vi "DefineColorPalette.vi"(10 "Files in":T2[](array[typedef]), 11 "FileList":refnum<vi>) -> (2 "Files out":T2[](array[typedef]))   [LabVIEW 2022 SP3]
uses:
  Curtin1_Label.ctl
panel:
  in  "new name":T1
  in  "Delete":bool
  in  "Clear":bool
  in  "Save":bool
  in  "Save as":bool
  in  "Apply":bool
  in  "Your Color Palettes":u16(ring) items=["Last Saved", "24 Colors", "fred", "rear"]
  in  "Colors":u32[](array[colorbox])
  # "Enter Color Name"
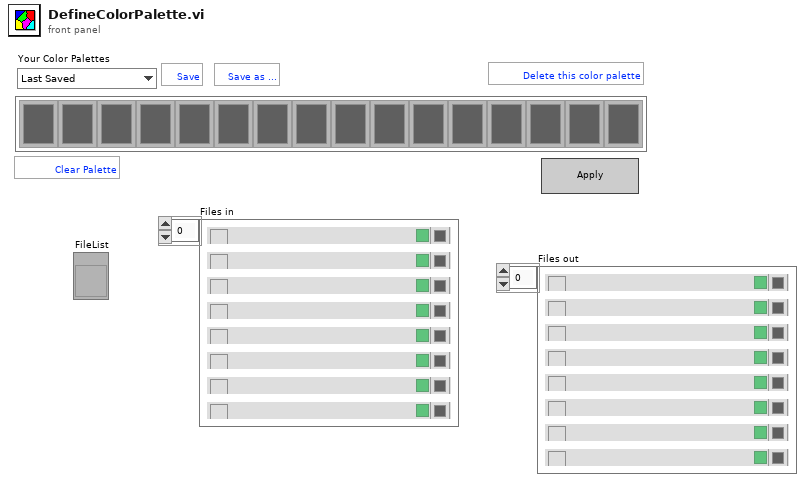
[diagram p1: front panel]
types:
  T1 = cluster{"Color Name":string, "OK Button":bool, "Cancel Button":bool}
  T2 = typedef "Curtin1_Label.ctl" = cluster{"Show?":bool, "Name":string, "Color":u32, "Path":path, "Show Notes":bool, "correlate":bool}
  T3 = enum16{"big-endian, network order", "native, host order", "little-endian"}
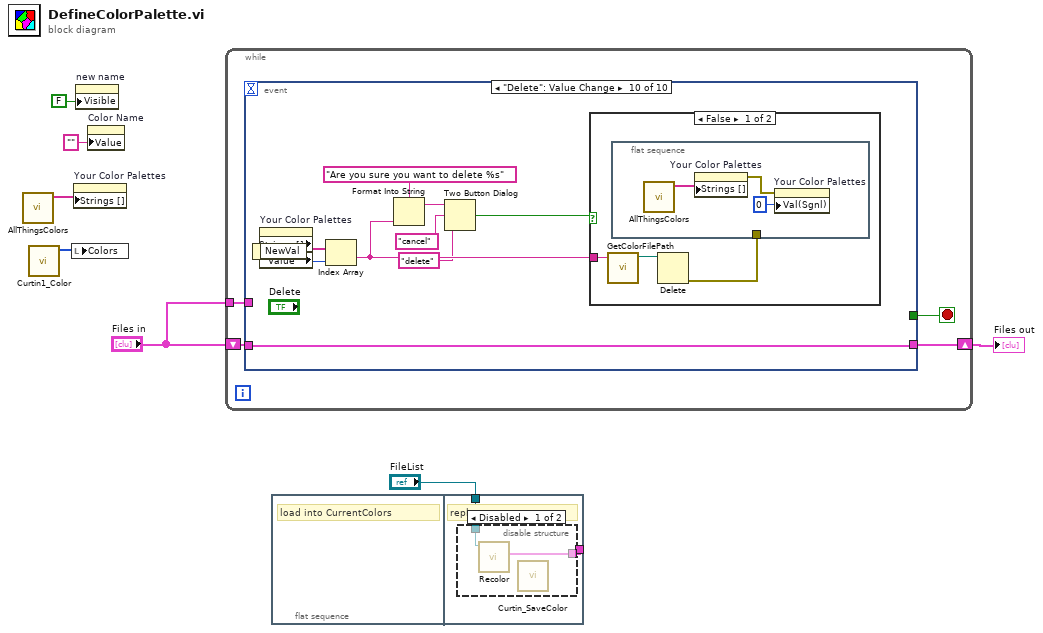
[diagram p0: block diagram]
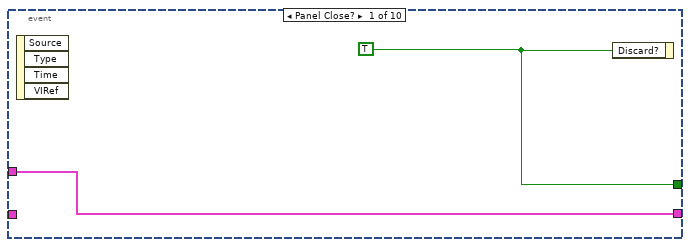
[diagram p3: hidden frame]
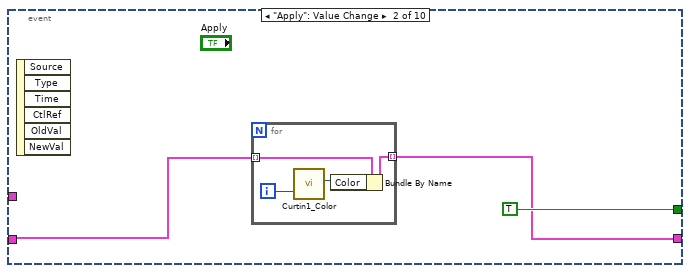
[diagram p4: hidden frame]
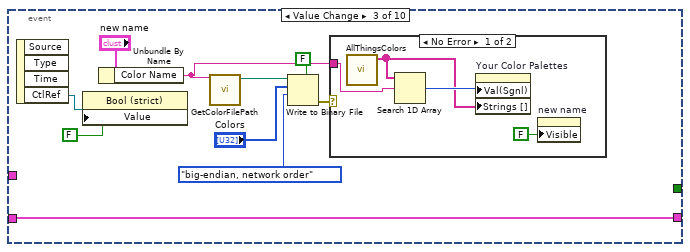
[diagram p5: hidden frame]
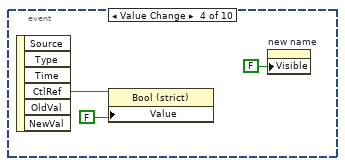
[diagram p7: hidden frame]
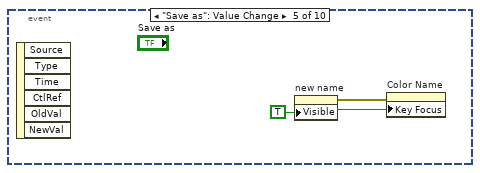
[diagram p8: hidden frame]
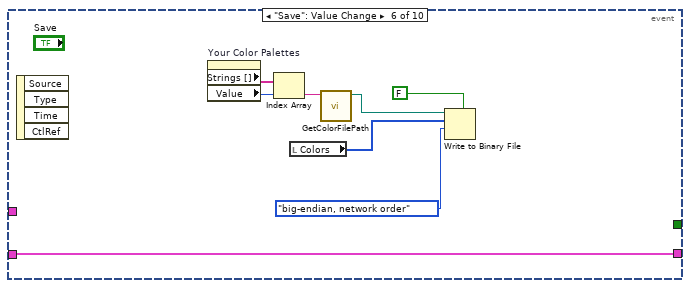
[diagram p9: hidden frame]
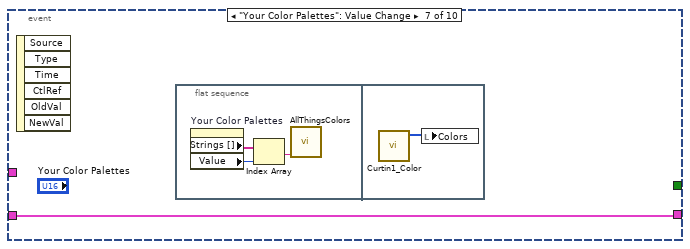
[diagram p10: hidden frame]
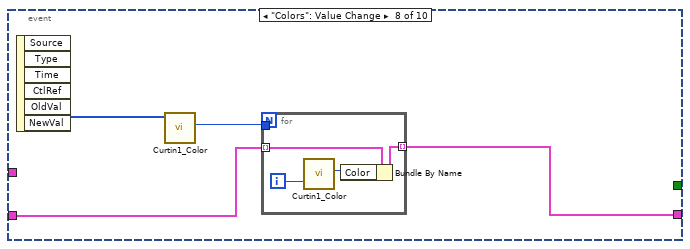
[diagram p11: hidden frame]
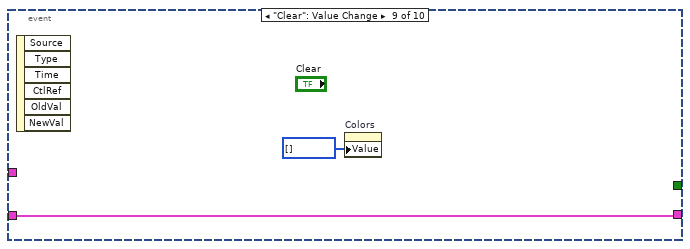
[diagram p12: hidden frame]
diagram:
  n1 = call "AllThingsColors.vi"() -> ("Possible Colors"=w7:string[])  [unwired: 11 in]
  n2 = call "Curtin1_Color.vi"() -> ("Color palette"=w3:u32[])  [unwired: 10 in, 1 out]
  n3 = local write "Colors"(w3) -> ()
  n4 = property on="Your Color Palettes" class="Ring (strict)"("Strings []"=w7) -> ()  [unwired: 2 in, 2 out]
  n5 = property on="new name" class="Clust (strict)"("Visible"=FALSE) -> ()  [unwired: 2 in, 2 out]
  n6 = property on="Color Name" class="Str"("Value"="") -> ()  [unwired: 2 in, 2 out]
  n7 = while {
    shift-right: [w10] -> w6
    shift-left: "Files in" -> [w9]
    tunnel: "Files in" -> [w8]
    stop <- w11 stop-if-true
    n8 = event shown="[9] \"Delete\": Value Change" {
      selector: _ -> [_ _ _ _ _ _ _ _ _ _]
      dyn-events: _ -> [_ _ _ _ _ _ _ _ _ _]
      timeout: _ -> [_ _ _ _ _ _ _ _ _ _]
      tunnel: [w13 TRUE ("Discard?") _ _ _ _ _ _ _ _] -> w11
      tunnel: [w12 w15 w30 _ _ w47 w48 w54 w62 w71] -> w10
      tunnel: w9 -> [_ w14 w30 _ _ w47 w48 w55 w62 w71]
      tunnel: w8 -> [w12 _ _ _ _ _ _ _ _ _]
      event Panel Close? {
        w13 = TRUE ("Discard?")
        n9 = event-data() -> ()  [unwired: 1 in, 4 out]
        n10 = event-data("Discard?"=w13) -> ()  [unwired: 1 in, 1 out]
      }
      event "Apply": Value Change {
        n11 = event-data() -> ()  [unwired: 1 in, 6 out]
        n12 = for {
          tunnel: w14 -> [w20] mode=indexing
          tunnel: [w19] -> w15 mode=indexing
          i -> [w18]
          n13 = call "Curtin1_Color.vi"("Offset"=w18) -> ("New color"=w17:u32)  [unwired: 9 in, 1 out]
          n14 = Bundle By Name(cluster=w20, "Color"=w17) -> (w19:T2)
        }
      }
      event "new name.OK Button": Value Change {
        n15 = event-data() -> ("CtlRef"=w21:refnum<vi>)  [unwired: 1 in, 3 out]
        n16 = property class="Bool (strict)"(reference=w21, "Value"=FALSE ("Visible")) -> ()  [unwired: 1 in, 2 out]
        n17 = Unbundle By Name("new name") -> ("Color Name"=w23:string)
        n18 = call "GetColorFilePath.vi"("String"=w23) -> ("path"=w25:path)  [unwired: 9 in, 1 out]
        n19 = Write to Binary File(file (use dialog)=w25, data="Colors", 5:FALSE ("prepend array or string size? (T)"), 9:T3."big-endian, network order" ("byte order (0:big-endian, network order)")) -> (error out=w26:errorcluster)  [unwired: 2 in, 2 out]
        n20 = case shown="No Error" w26 {
          tunnel: w23 -> [w34 _]
          frame No Error {
            n21 = call "AllThingsColors.vi"() -> ("Possible Colors"=w32:string[])  [unwired: 11 in]
            n22 = Search 1D Array(1D array=w32, element=w34) -> (index of element=w33:i32)  [unwired: 1 in]
            n23 = property on="Your Color Palettes" class="Ring (strict)"("Val(Sgnl)"=w33, "Strings []"=w32) -> ()  [unwired: 2 in, 2 out]
            n24 = property on="new name" class="Clust (strict)"("Visible"=FALSE) -> ()  [unwired: 2 in, 2 out]
          }
          frame Error {
          }
        }
      }
      event "new name.Cancel Button": Value Change {
        n25 = event-data() -> ("CtlRef"=w36:refnum<vi>)  [unwired: 1 in, 5 out]
        n26 = property class="Bool (strict)"(reference=w36, "Value"=FALSE ("Visible")) -> ()  [unwired: 1 in, 2 out]
        n27 = property on="new name" class="Clust (strict)"("Visible"=FALSE) -> ()  [unwired: 2 in, 2 out]
      }
      event "Save as": Value Change {
        w38 = TRUE ("Visible")
        n28 = event-data() -> ()  [unwired: 1 in, 6 out]
        n29 = property on="new name" class="Clust (strict)"("Visible"=w38) -> (error out=w39:errorcluster)  [unwired: 2 in, 1 out]
        n30 = property on="Color Name" class="Str"(error in=w39, "Key Focus"=w38) -> ()  [unwired: 1 in, 2 out]
      }
      event "Save": Value Change {
        n31 = event-data() -> ()  [unwired: 1 in, 4 out]
        n32 = property on="Your Color Palettes" class="Ring (strict)"() -> ("Strings []"=w41:string[], "Value"=w42:u16)  [unwired: 2 in, 2 out]
        n33 = Index Array(array=w41, index=w42) -> (element=w40:string)
        n34 = local read "Colors"() -> (w43:u32[])
        n35 = call "GetColorFilePath.vi"("String"=w40) -> ("path"=w44:path)  [unwired: 9 in, 1 out]
        n36 = Write to Binary File(file (use dialog)=w44, data=w43, 5:FALSE ("prepend array or string size? (T)"), 9:T3."big-endian, network order" ("byte order (0:big-endian, network order)")) -> ()  [unwired: 2 in, 3 out]
      }
      event "Your Color Palettes": Value Change {
        n37 = event-data() -> ()  [unwired: 1 in, 6 out]
        n38 = flat-sequence {
          frame #0 {
            n39 = property on="Your Color Palettes" class="Ring (strict)"() -> ("Strings []"=w50:string[], "Value"=w49:u16)  [unwired: 2 in, 2 out]
            n40 = Index Array(array=w50, index=w49) -> (element=w51:string)
            n41 = call "AllThingsColors.vi"("Choice"=w51) -> ()  [unwired: 10 in, 1 out]
          }
          frame #1 {
            n42 = call "Curtin1_Color.vi"() -> ("Color palette"=w52:u32[])  [unwired: 10 in, 1 out]
            n43 = local write "Colors"(w52) -> ()
          }
        }
      }
      event "Colors": Value Change {
        n44 = event-data() -> ("NewVal"=w56:u32[])  [unwired: 1 in, 5 out]
        n45 = call "Curtin1_Color.vi"("Color"=w56) -> ("New color"=w53:u32)  [unwired: 9 in, 1 out]
        n46 = for {
          tunnel: w55 -> [w60] mode=indexing
          tunnel: [w59] -> w54 mode=indexing
          tunnel: w53 -> [_]
          i -> [w58]
          n47 = call "Curtin1_Color.vi"("Offset"=w58) -> ("New color"=w57:u32)  [unwired: 9 in, 1 out]
          n48 = Bundle By Name(cluster=w60, "Color"=w57) -> (w59:T2)
        }
      }
      event "Clear": Value Change {
        n49 = event-data() -> ()  [unwired: 1 in, 6 out]
        n50 = property on="Colors" class="Arr (strict)"("Value"=u32[] [] ("Colors")) -> ()  [unwired: 2 in, 2 out]
      }
      event "Delete": Value Change {
        n51 = event-data() -> ()  [unwired: 1 in, 1 out]
        n52 = property on="Your Color Palettes" class="Ring (strict)"() -> ("Strings []"=w69:string[], "Value"=w70:u16)  [unwired: 2 in, 2 out]
        n53 = Index Array(array=w69, index=w70) -> (element=w67:string)
        n54 = Format Into String(format string="Are you sure you want to delete %s", w67) -> (resulting string=w66:string)  [unwired: 2 in, 1 out]
        n55 = Two Button Dialog(message=w66, 1:"delete" ("F button name (\"Cancel\")"), 2:"cancel" ("T button name (\"OK\")")) -> (T button?=w63:bool)
        n56 = case shown="False" w63 {
          tunnel: w67 -> [w74 _]
          frame False {
            n57 = call "GetColorFilePath.vi"("String"=w74) -> ("path"=w73:path)  [unwired: 9 in, 1 out]
            n58 = flat-sequence {
              tunnel: w72 -> [_]
              frame #0 {
                n59 = call "AllThingsColors.vi"() -> ("Possible Colors"=w76:string[])  [unwired: 11 in]
                n60 = property on="Your Color Palettes" class="Ring (strict)"("Strings []"=w76) -> (error out=w75:errorcluster)  [unwired: 2 in, 1 out]
                n61 = property on="Your Color Palettes" class="Ring (strict)"(error in=w75, "Val(Sgnl)"=0) -> ()  [unwired: 1 in, 2 out]
              }
            }
            n62 = Delete(path (use dialog)=w73) -> (error out=w72:errorcluster)  [unwired: 4 in, 2 out]
          }
          frame True {
          }
        }
      }
    }
  }
  "Files out" <- w6
  n63 = flat-sequence {
    tunnel: "FileList" -> [w79]
    tunnel: [w78] -> _
    frame #0 {
      # "load into CurrentColors"
    }
    frame #1 {
      # "replot"
      n64 = disable-structure shown="Disabled" {
        disable-tunnel: w79 -> [w81 _]
        disable-tunnel: [w80 _] -> w78
        frame Disabled {
          n65 = call "Recolor.vi"("Array in"=w81) -> ("Files"=w80:T2[])  [unwired: 10 in]
          n66 = call "Curtin_SaveColor.vi"() -> ()  [unwired: 10 in, 2 out]
        }
        frame Enabled {
        }
      }
    }
  }
